vi "GPS Reached waypoint.vi"(7 "Required distance to target (meters)":dbl, 8 "Number of WP Reached IN":i8, 10 "Current Co-ordinates":T1 {"Longitude" format="%#_14g"; "Latitude" format="%#_14g"}, 11 "Waypoint List In":T1[](array[typedef]) {"Longitude" format="%#_14g"; "Latitude" format="%#_14g"}) -> (0 "Number of WP Reached OUT":i8, 2 "Reached waypoint?":bool, 3 "Waypoint List Out":T1[](array[typedef]) {"Longitude" format="%#_14g"; "Latitude" format="%#_14g"}, 4 "Distance to Target (meters)":dbl=0.5)   [LabVIEW 2009]
uses:
  TypeDefs/Sensor TypeDefs/GPS Data.ctl
  <vilib>/userDefined/High Color/nirio_resource_hc.ctl
  <vilib>/rvi/interface/nirviOpenFPGA/nirviOpenFPGA.xnode
  FPGA Bitfiles/Q_IGVC_2010.lvproj_FPGA Target_FPGA_MAIN.vi.lvbitx
  <vilib>/FPGAPlugInAG/cRIO-9113/nirviIntfOpen_cRIO-9113.vi
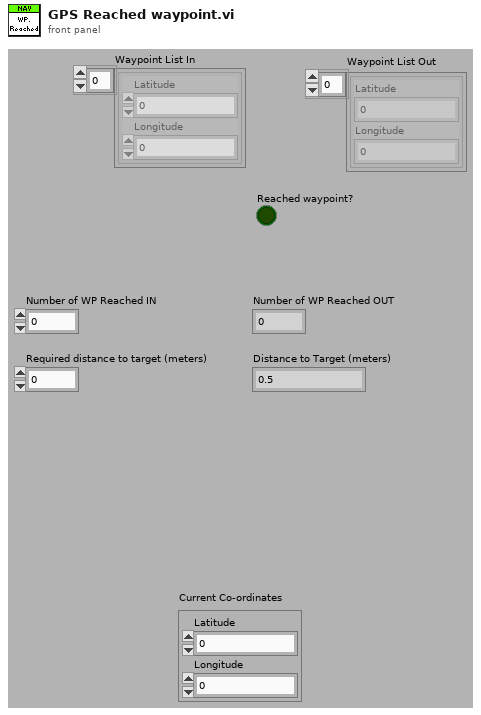
[diagram p1: front panel]
types:
  T1 = typedef "GPS Data.ctl" = cluster{"Latitude":dbl, "Longitude":dbl}
  T2 = typedef "nirio_resource_hc.ctl" = tag
  T3 = cluster{"signature":u8[], "vi signatures match":bool, "signature register address":u32, "reset register address":u32, "control register address":u32, "interrupt base address":u32, "Bitstream Version":u32, "DMA Configuration":cluster{"Name":string, "Depth":u32, "Write? (Deprecated:Use Implementation)":bool, "Physical Channel":u32, "Base Address":u32, "Data Width":u32, "Data Type":enum32{"Boolean", "I8", "I16", "I32", "I64", "U8", "U16", "U32", "U64", "FXP"}, "FXP Properties":variant, "Write Window Address":u32, "Implementation":enum16{"niFpgaTargetToHost", "niFpgaHostToTarget", "niFpgaPeerToPeerWriter", "niFpgaPeerToPeerReader", "niCoreTargetToHost", "niCoreHostToTarget"}, "Control Set":u32}[], "run when loaded?":bool, "reset register size in bits":u32, "compilation results xml":string}
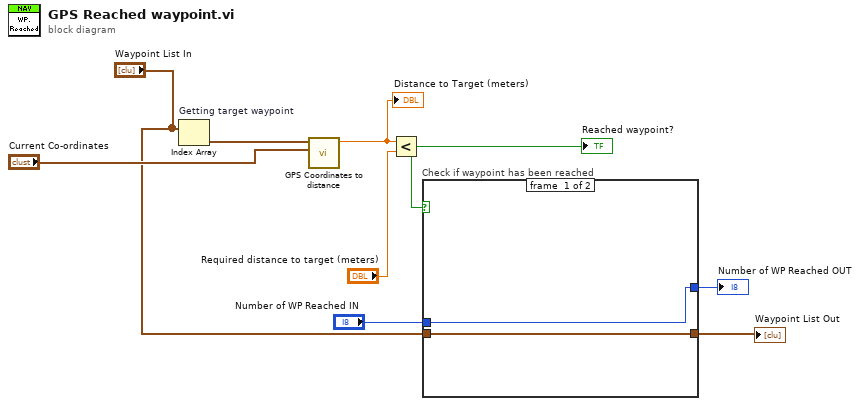
[diagram p0: block diagram]
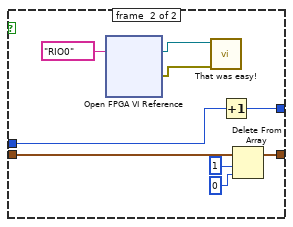
[diagram p2: hidden frame]
diagram:
  n1 = Index Array "Getting target waypoint"(array="Waypoint List In") -> (element=w5:T1)  [unwired: 1 in]
  n2 = call "GPS Coordinates to distance.vi"("GPS Co-ordinate 2"="Current Co-ordinates", "GPS Co-ordinate 1"=w5) -> ("Distance"=w4:dbl)  [unwired: 9 in]
  "Distance to Target (meters)" <- w4
  n3 = Less?(x=w4, y="Required distance to target (meters)") -> (x < y?=w9:bool)
  "Reached waypoint?" <- w9
  n4 = case "Check if waypoint has been reached" shown="True" w9 {
    tunnel: "Waypoint List In" -> [w11 w20]
    tunnel: [w11 w17] -> w1
    tunnel: [w10 w16] -> w7
    tunnel: "Number of WP Reached IN" -> [w10 w15]
    frame #0 {
    }
    frame #1 {
      n5 = xnode "Open FPGA VI Reference"("resource name"=T2 "RIO0") -> ("FPGA VI Reference Out"=w13:refnum<k20>, "error out"=w12:errorcluster)  [unwired: 1 in]
      n6 = call "That was easy!.vi"("error in (no error)"=w12, "FPGA VI Reference in"=w13) -> ()  [unwired: 8 in, 2 out]
      n7 = Increment(x=w15) -> (x+1=w16:i8)
      n8 = Delete From Array(array=w20, length=1, index=0) -> (array with subset deleted=w17:T1[])  [unwired: 1 out]
    }
  }
  "Number of WP Reached OUT" <- w7
  "Waypoint List Out" <- w1
